vi "Piston.vi"(11 "Robot Commands":T1) -> ()   [LabVIEW 2015]
uses:
  Joystick/Robot Commands.ctl
  <vilib>/Rock Robotics/WPI/Solenoid/WPI_SolenoidValue.ctl
  Global Variables/Refnum Names.vi
  <vilib>/Rock Robotics/WPI/Solenoid/WPI_SolenoidSetEnum.vi
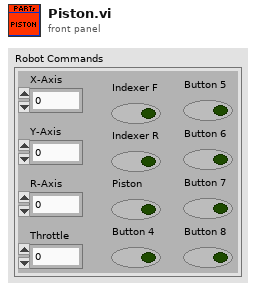
[diagram p1: front panel]
types:
  T1 = typedef "Robot Commands.ctl" = cluster{"X-Axis":dbl, "Y-Axis":dbl, "R-Axis":dbl, "Throttle":dbl, "Indexer F":bool, "Indexer R":bool, "Piston":bool, "Button 4":bool, "Button 5":bool, "Button 6":bool, "Button 7":bool, "Button 8":bool}
  T2 = typedef "WPI_SolenoidValue.ctl" = enum16{"Off", "On", "Forward", "Reverse"}
  T3 = typedef "WPI_SolenoidDevRef.ctl" = cluster{"DevStatus":errorcluster, "Pneumatics Control Module":u8, "Forward Solenoid Channel":T4, "Reverse Solenoid Channel":T4}
  T4 = typedef "WPI_SolenoidChannel.ctl" = enum8{"Solenoid 0", "Solenoid 1", "Solenoid 2", "Solenoid 3", "Solenoid 4", "Solenoid 5", "Solenoid 6", "Solenoid 7", "Invalid"}
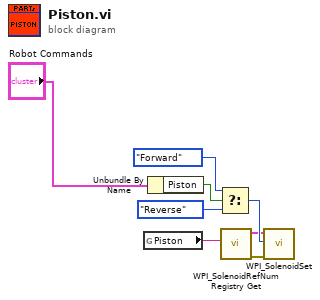
[diagram p0: block diagram]
diagram:
  n1 = global read "Refnum Names.vi" "Piston"() -> (w5:string)
  n2 = Unbundle By Name("Robot Commands") -> ("Piston"=w1:bool)
  n3 = Select(t=WPI_SolenoidValue."Forward" ("Value"), s=w1, f=WPI_SolenoidValue."Reverse" ("Value")) -> (s? t:f=w7:T2)
  n4 = call <vilib>:"WPI_SolenoidRefNum Registry Get.vi"("refnum name"=w5) -> ("error out"=w6:errorcluster, "SolenoidDevRef"=w4:T3)  [unwired: 9 in]
  n5 = call-poly <vilib>:"WPI_SolenoidSet.vi"("error in (no error)"=w6, "Value"=w7, "SolenoidDevRef"=w4) -> ()  [unwired: 7 in, 2 out]
